vi "Execute Query.vi"(8 "error in (no error)":errorcluster, 10 "Query":string, 11 "SLL Database in":refnum<class "SLL Database.lvclass">) -> (0 "error out":errorcluster, 2 "Data Output":string[][](array[string]), 3 "SLL Database out":refnum<class "SLL Database.lvclass">)   [LabVIEW 2014, in "SLL Database.lvclass"]
uses:
  SLL Database.lvclass
  SLL Database.lvclass/SLL Database.ctl
  <vilib>/addons/database/Connection.llb/Conn Execute.vi
  <vilib>/addons/database/Recordset.llb/Rec Fetch Recordset Data (R).vi
  <vilib>/addons/database/Recordset.llb/Rec Destroy - Connection.vi
  <vilib>/addons/database/NI_Database_API.lvlib
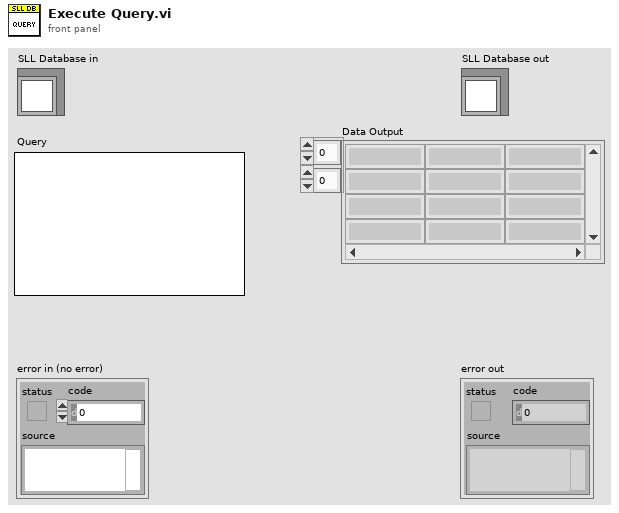
[diagram p1: front panel]
types:
  T1 = typedef "NI_Database_API.lvlib/Conn ObjectReference.ctl" = refnum<k1>
  T2 = typedef "NI_Database_API.lvlib/Rec ObjectReference.ctl" = refnum<k1>
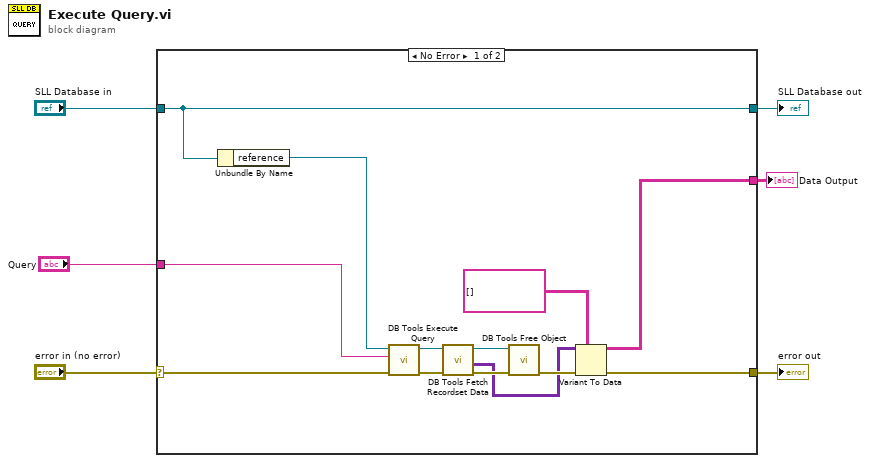
[diagram p0: block diagram]
diagram:
  n1 = case shown="No Error" "error in (no error)" {
    selector: "error in (no error)" -> [w19 w21]
    tunnel: [w11 w21] -> w5
    tunnel: [w18 w20] -> w3
    tunnel: "SLL Database in" -> [w18 w20]
    tunnel: [w8 _] -> w2
    tunnel: "Query" -> [w7 _]
    frame No Error {
      n2 = Unbundle By Name(w18) -> ("reference"=w12:T1)
      n3 = call-poly <vilib>:"DB Tools Execute Query.vi"("error in (no error)"=w19, "SQL query"=w7, "connection reference"=w12) -> ("error out"=w17:errorcluster, "recordset reference"=w14:T2)  [unwired: 5 in]
      n4 = call-poly <vilib>:"DB Tools Fetch Recordset Data.vi"("error in (no error)"=w17, "recordset reference"=w14) -> ("error out"=w16:errorcluster, "recordset data"=w10:variant[][], "recordset reference out"=w13:T2)  [unwired: 3 in]
      n5 = call-poly <vilib>:"DB Tools Free Object.vi"("error in (no error)"=w16, "recordset reference"=w13) -> ("error out"=w15:errorcluster)  [unwired: 8 in, 1 out]
      n6 = Variant To Data(error in=w15, type=string[][] [], Variant=w10) -> (data=w8:string[][], error out=w11:errorcluster)
    }
    frame Error {
    }
  }
  "error out" <- w5
  "SLL Database out" <- w3
  "Data Output" <- w2
